vi "seleccionarEquipo.vi"(8 "error in (no error)":errorcluster) -> (0 "error out":errorcluster, 2 "Equipo.lvclass":refnum<class "Equipo.lvclass">, 3 "Fabrica de Equipo out":refnum<class "Fabrica de Equipos.lvclass">)   [LabVIEW 2019, in "Fabrica de Equipos.lvclass"]
uses:
  Fabrica de Equipos.lvclass
  Equipo/Equipo.lvclass
  Sonometro/Sonometro.lvclass
  C:/Users/ivan_/Documents/procal/Equipo/Equipo/Equipo.lvclass
  Dosimetro/Dosimetro.lvclass
  Calibrador/Calibrador.lvclass
  Fabrica de Equipos.lvclass/Fabrica de Equipos.ctl
panel:
  in  "Calibrador":bool
  in  "Dosimetro":bool
  in  "Sonometro":bool
  # "Seleccione el equipo a calibrar"
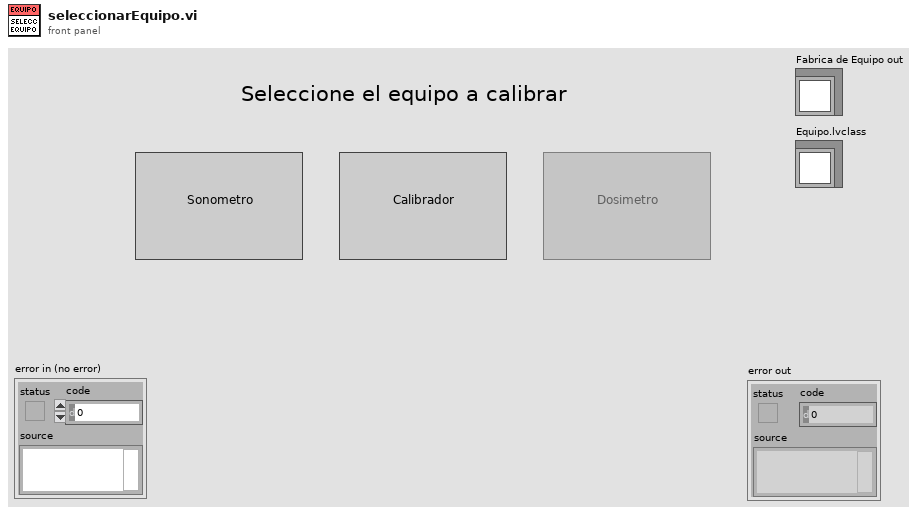
[diagram p1: front panel]
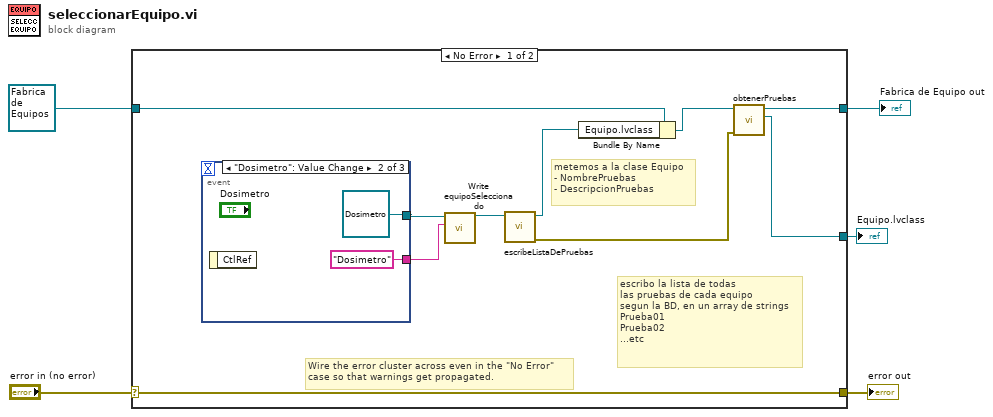
[diagram p0: block diagram]
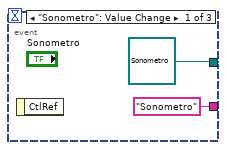
[diagram p2: hidden frame]
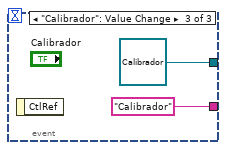
[diagram p3: hidden frame]
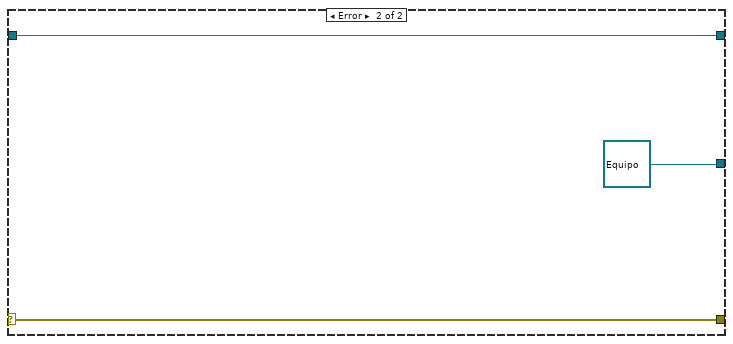
[diagram p4: hidden frame]
diagram:
  n1 = case shown="No Error" "error in (no error)" {
    selector: "error in (no error)" -> [w15 w24]
    tunnel: [w15 w24] -> w4
    tunnel: refnum<class "Fabrica de Equipos.lvclass"> refnum ("Equipo in") -> [w14 w23]
    tunnel: [w10 w23] -> w2
    tunnel: [w9 refnum<class "Equipo.lvclass"> refnum ("Equipo.lvclass")] -> w1
    frame No Error {
      # "escribo la lista de todas\nlas pruebas de cada equipo\nsegun la BD, en un array de strings\nPrueba01\nPrueba02\n...etc"
      # "metemos a la clase Equipo\n- NombrePruebas\n- DescripcionPruebas"
      # "Wire the error cluster across even in the \"No Error\"\ncase so that warnings get propagated."
      n2 = event shown="[1] \"Dosimetro\": Value Change" {
        selector: _ -> [_ _ _]
        dyn-events: _ -> [_ _ _]
        timeout: _ -> [_ _ _]
        tunnel: [refnum<class "Sonometro.lvclass"> refnum ("Sonometro.lvclass") refnum<class "Dosimetro.lvclass"> refnum ("Dosimetro.lvclass") refnum<class "Calibrador.lvclass"> refnum ("Calibrador.lvclass")] -> w8
        tunnel: ["Sonometro" "Dosimetro" "Calibrador"] -> w6
        event "Sonometro": Value Change {
          n3 = event-data() -> ()  [unwired: 1 in, 1 out]
        }
        event "Dosimetro": Value Change {
          n4 = event-data() -> ()  [unwired: 1 in, 1 out]
        }
        event "Calibrador": Value Change {
          n5 = event-data() -> ()  [unwired: 1 in, 1 out]
        }
      }
      n6 = call-dynamic "Write equipoSeleccionado.vi"("equipoSeleccionado"=w6, "Equipo in"=w8) -> ("Equipo out"=w7:refnum<class "Equipo.lvclass">)  [unwired: 8 in, 1 out]
      n7 = call-dynamic "escribeListaDePruebas.vi"("Equipo in"=w7) -> ("error out"=w11:errorcluster, "Equipo out"=w13:refnum<class "Equipo.lvclass">)  [unwired: 9 in]
      n8 = Bundle By Name(cluster=w14, "Equipo.lvclass"=w13) -> (w12:refnum<class "Fabrica de Equipos.lvclass">)
      n9 = call "obtenerPruebas.vi"("error in (no error)"=w11, "Equipo in"=w12) -> ("Equipo.lvclass"=w9:refnum<class "Equipo.lvclass">, "Equipo out"=w10:refnum<class "Fabrica de Equipos.lvclass">)  [unwired: 7 in, 1 out]
    }
    frame Error {
    }
  }
  "error out" <- w4
  "Fabrica de Equipo out" <- w2
  "Equipo.lvclass" <- w1
